vi "cont_array.vi"(8 "edge_cluster":cluster{"Array":sgl[], "Array":bool[]}, 11 "u8_ar_phase map":u8[](array[numeric])) -> (3 "Array":i16[](array[numeric]))   [LabVIEW 2011]
panel:
  out "Boolean":bool
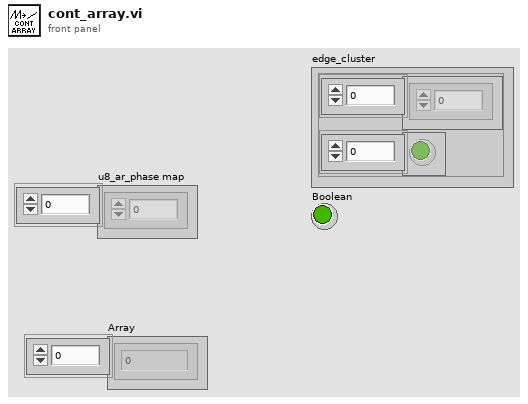
[diagram p1: front panel]
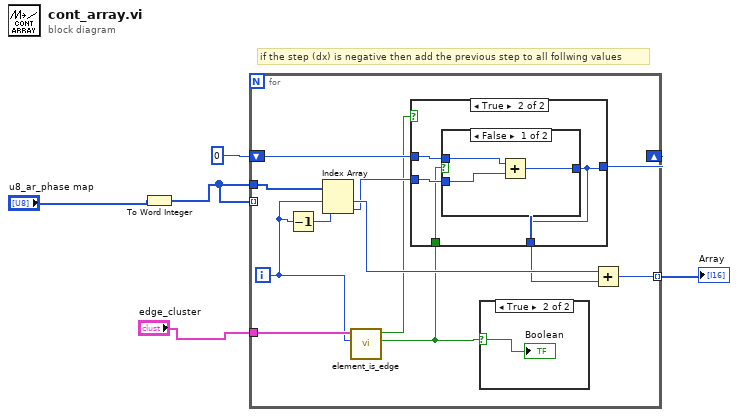
[diagram p0: block diagram]
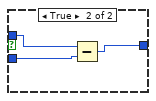
[diagram p4: hidden frame]
diagram:
  # "if the step (dx) is negative then add the previous step to all follwing values"
  n1 = To Word Integer(number="u8_ar_phase map") -> (16bit integer=w2:i16[])
  n2 = for {
    tunnel: w2 -> [w17]
    tunnel: w2 -> [_] mode=indexing
    shift-right: [w14] -> _
    shift-left: i16 0 -> [w13]
    tunnel: [w11] -> w4 mode=indexing
    tunnel: "edge_cluster" -> [w10]
    i -> [w9]
    n3 = Decrement(x=w9) -> (x-1=w8:i32)
    n4 = Index Array(array=w17, index #1=w9, index #2=w8) -> (element #1=w16:i16, element #2=w15:i16)
    n5 = call "element_is_edge.vi"("current element"=w9, "edge_cluster"=w10) -> ("direction (rising/falling)"=w6:bool, "edge"=w7:bool)  [unwired: 8 in]
    n6 = case shown="True" w7 {
      tunnel: w15 -> [_ w23]
      tunnel: [w19 w21] -> w14
      tunnel: w13 -> [w19 w22]
      tunnel: [w19 w21] -> w12
      tunnel: w6 -> [_ w20]
      frame False {
      }
      frame True {
        n7 = case shown="False" w20 {
          tunnel: w23 -> [w26 w28]
          tunnel: w22 -> [w25 w29]
          tunnel: [w24 w27] -> w21
          frame False {
            n8 = Add(x=w25, y=w26) -> (x+y=w24:i16)
          }
          frame True {
            n9 = Subtract(x=w29, y=w28) -> (x-y=w27:i16)
          }
        }
      }
    }
    n10 = case shown="True" w6 {
      selector: w6 -> [_ w18]
      frame False {
      }
      frame True {
        "Boolean" <- w18
      }
    }
    n11 = Add(x=w16, y=w12) -> (x+y=w11:i16)
  }
  "Array" <- w4
